vi "SpaceX Main.vi"() -> ()   [LabVIEW 2022 SP3]
uses:
  AppData/Local/Temp/703aeb86-a1ff-4ba8-9387-38d48ae470f4_SpaceX Demo.zip.0f4/SpaceX Demo/SubVIs/States.ctl
  <vilib>/LabVIEW Interface for Arduino/Type Defs/Pin Mode.ctl
panel:
  in  "Dragon Capsule Delay Time (s)":dbl=1.0 caption="Delay Time (s)"
  in  "Wave Delay (s)":dbl=1.0 caption="Delay Time (s)"
  in  "Rocket Launch Delay Time (s)":dbl caption="Delay Time (s)"
  in  "Rocket Launch Motor Pin":u8=3
  in  "Dragon Capsule Motor Pin":u8=11
  in  "Rocket Motor Speed":u8=100
  in  "Dragon Capsule Speed":u8=50
  in  "Reset Mode":bool
  in  "Rocket Backwards":bool
  in  "Capsule Backwards":bool
  out "Demo Ready?":bool
  out "Hall Effect Sensor Value":dbl
  in  "Rocket Launch Complete":bool
  in  "GO Button":bool
  in  "stop":bool
  in  "Kinect Close Button":bool
  in  "Launch Pad Pin":u8=5
  in  "Wave Pins":T1={"Wave 1 Pin"=6, "Wave 2 Pin"=7, "Wave 3 Pin"=8, "Wave 4 Pin"=9, "Wave 5"=10}
  out "State Machine: Current State":T2
  in  "Pulse Speed":u8(knob)=3 scale=1.0..10.0
  out "Launch Pad Voltage Level":dbl(knob) scale=0.0..255.0
  in  "Number of Pulses":i32=4
  in  "stop 2":bool
  # "Delay Settings"
  # "Motor Configuration"
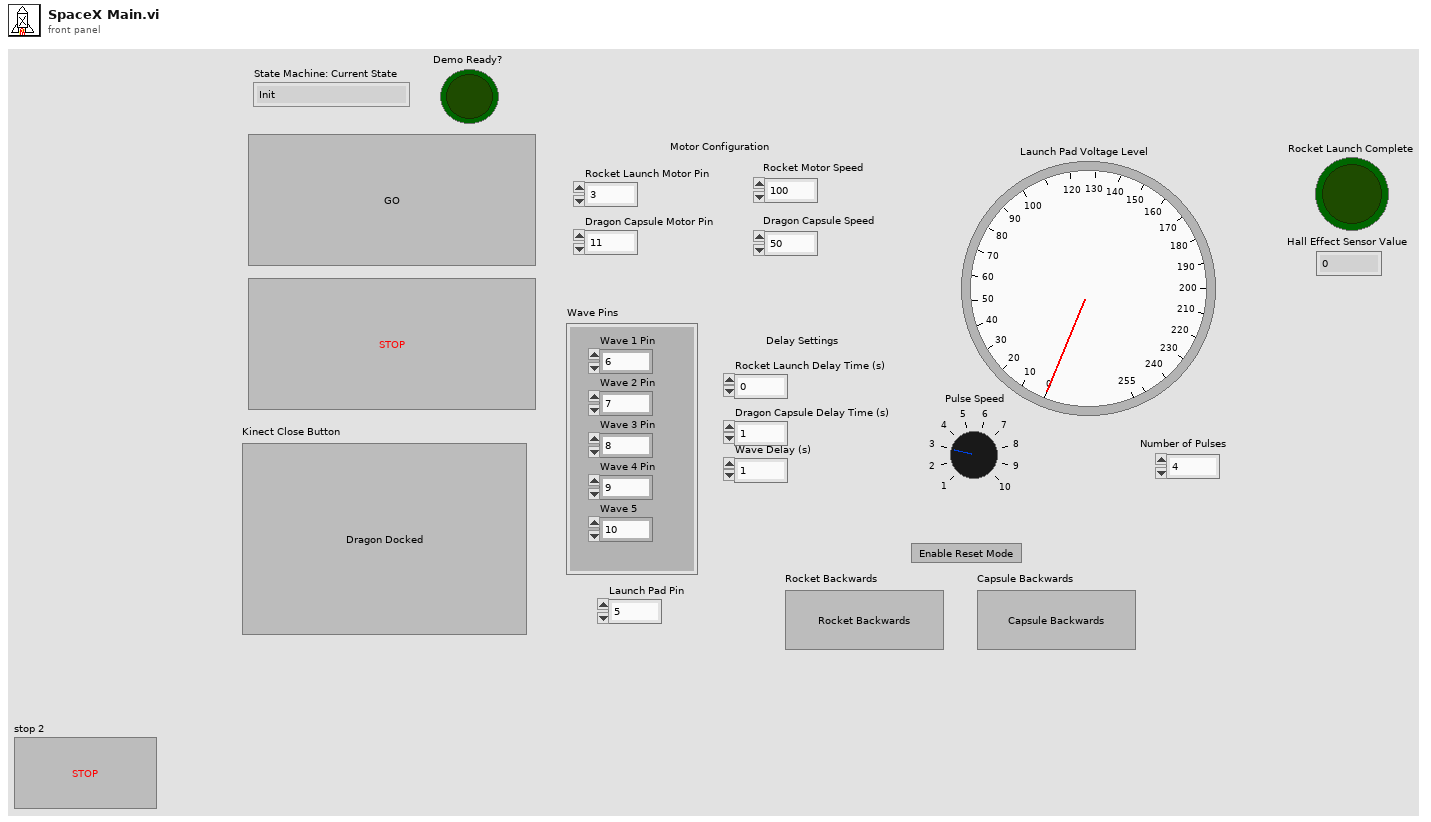
[diagram p1: front panel]
types:
  T1 = cluster{"Wave 1 Pin":u8, "Wave 2 Pin":u8, "Wave 3 Pin":u8, "Wave 4 Pin":u8, "Wave 5":u8}
  T2 = typedef "States.ctl" = enum16{"Init", "Run", "Shutdown", "Rocket Launch", "Dragon Travel", "Communicate", "Reset"}
  T3 = typedef "LabVIEW Interface for Arduino.lvlib/Pin Mode.ctl" = enum8{"Input", "Output"}
  T4 = typedef "LabVIEW Interface for Arduino.lvlib/Arduino Resource.ctl" = cluster{"VISA resource":refnum<visa-resource-name>, "Board Type":T5, "Connection Type":enum8{"USB / Serial"}, "Bytes Per Packet (15)":u8}
  T5 = typedef "LabVIEW Interface for Arduino.lvlib/Board Type.ctl" = enum16{"Uno", "Dimuelanove w/Atmega 328", "Mega 2560"}
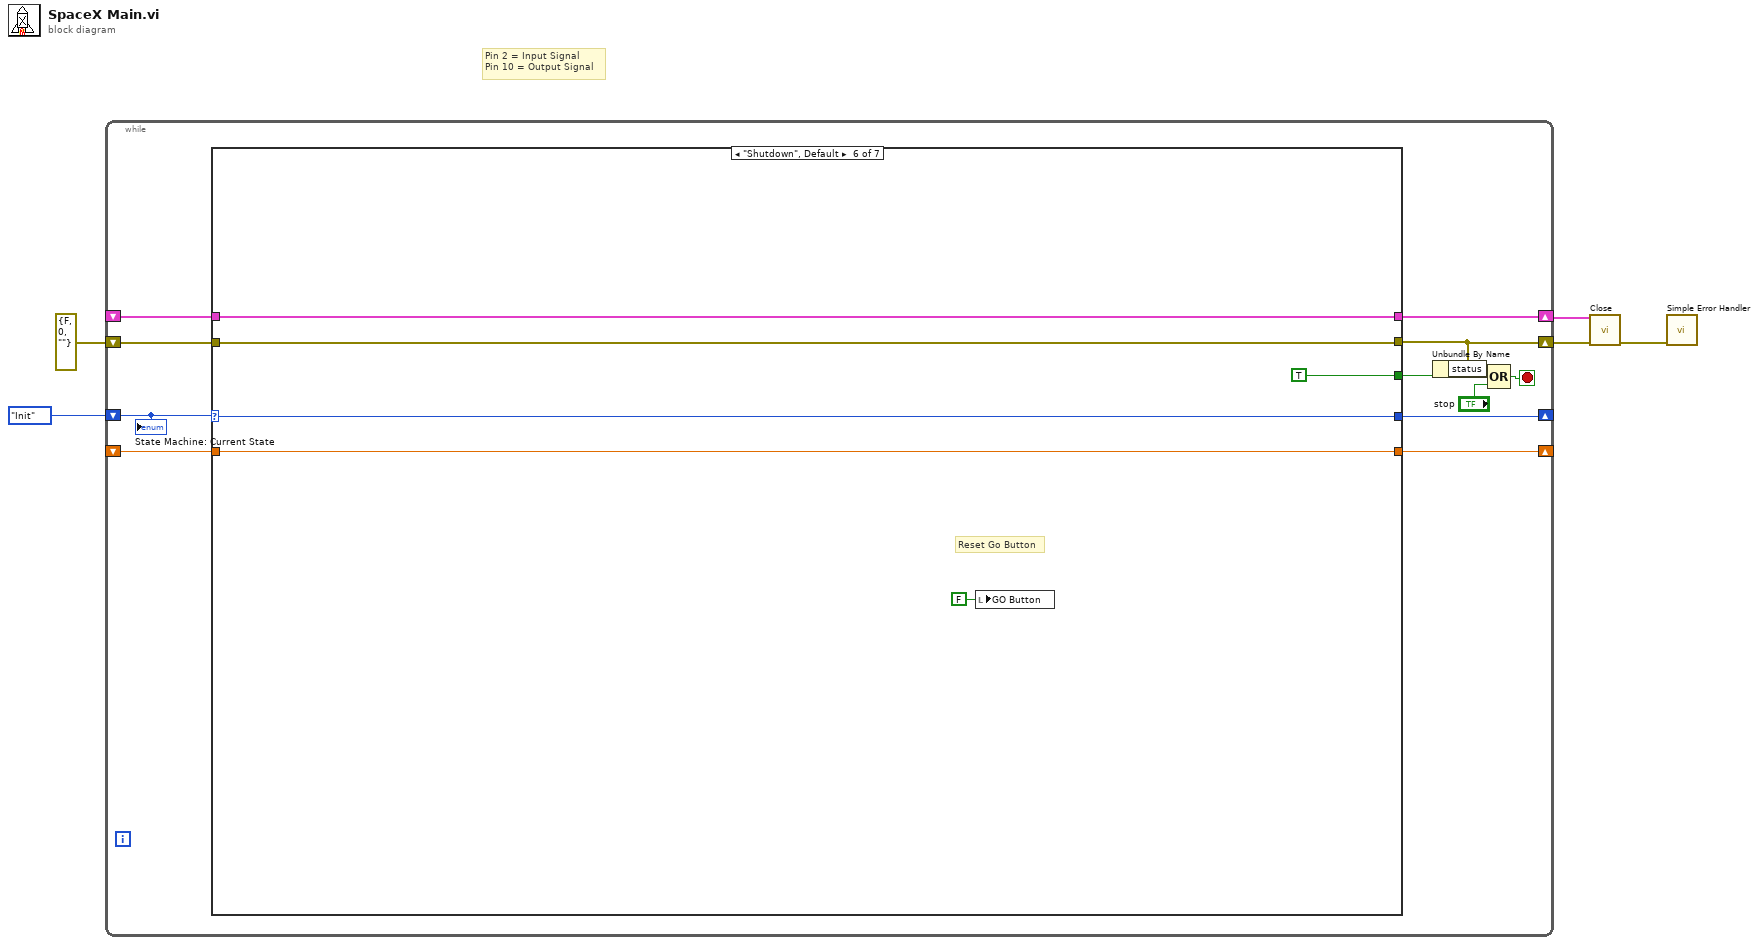
[diagram p0: block diagram]
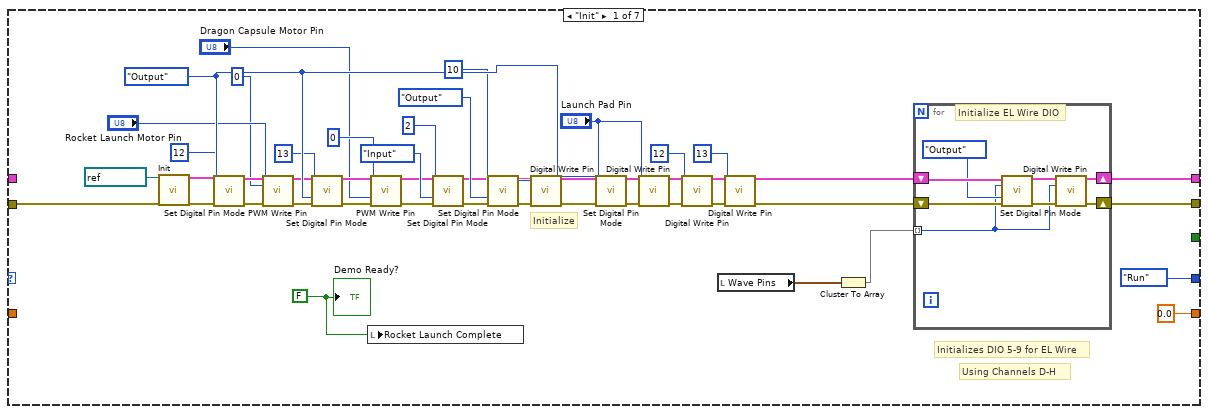
[diagram p2: hidden frame]
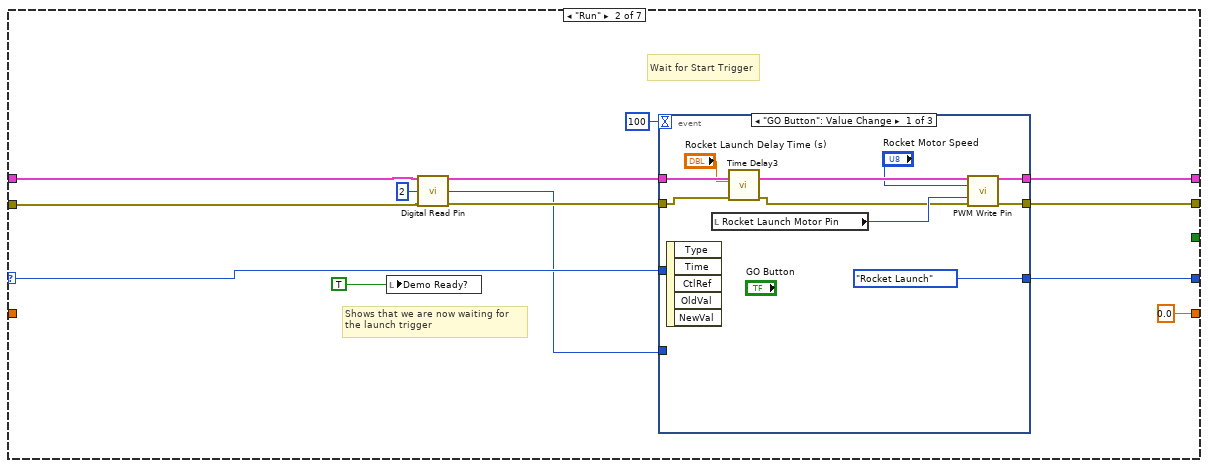
[diagram p3: hidden frame]
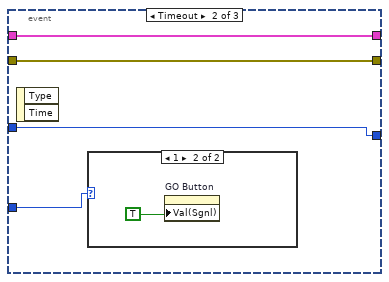
[diagram p4: hidden frame]
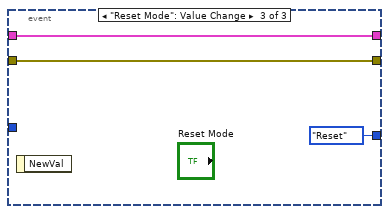
[diagram p6: hidden frame]
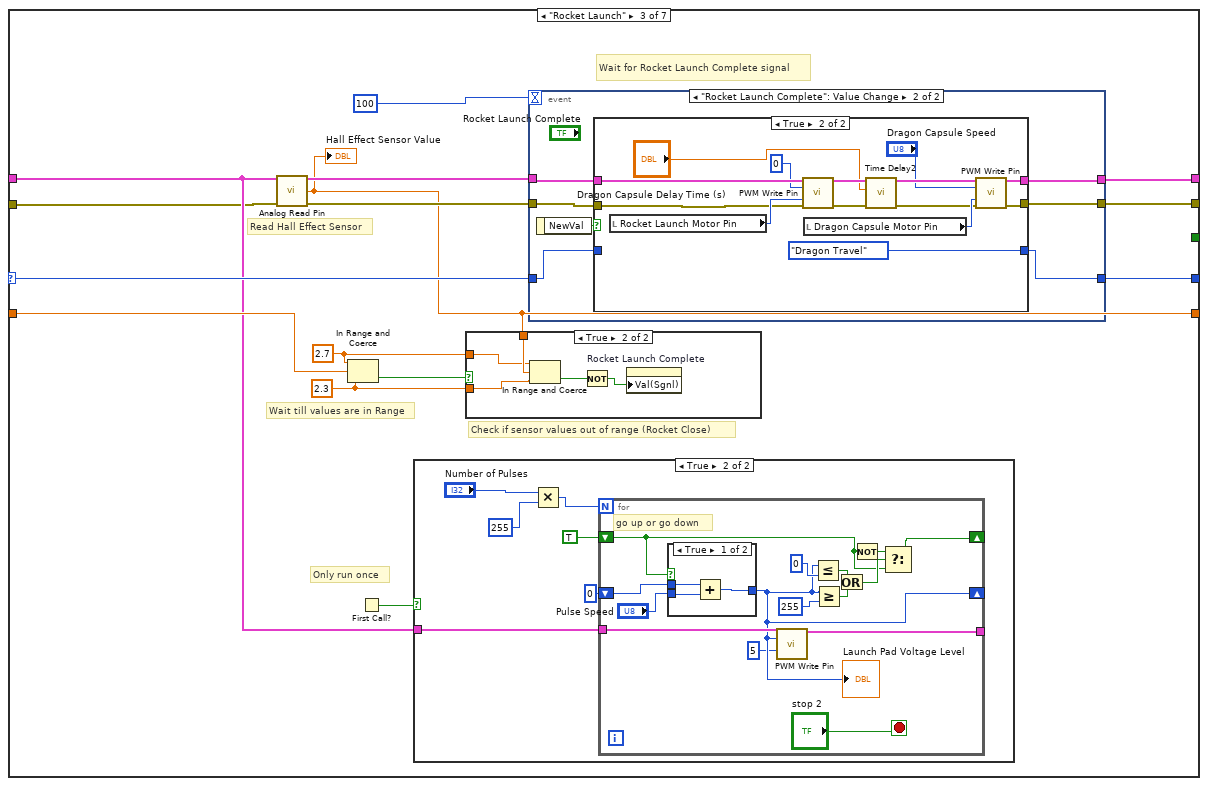
[diagram p7: hidden frame]
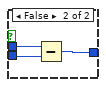
[diagram p9: hidden frame]
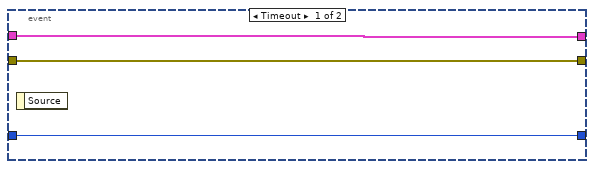
[diagram p11: hidden frame]
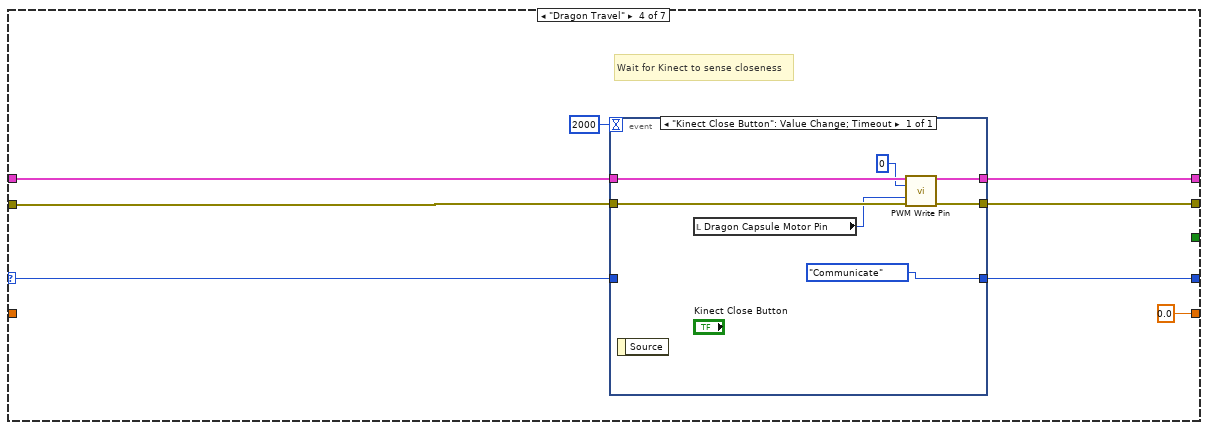
[diagram p13: hidden frame]
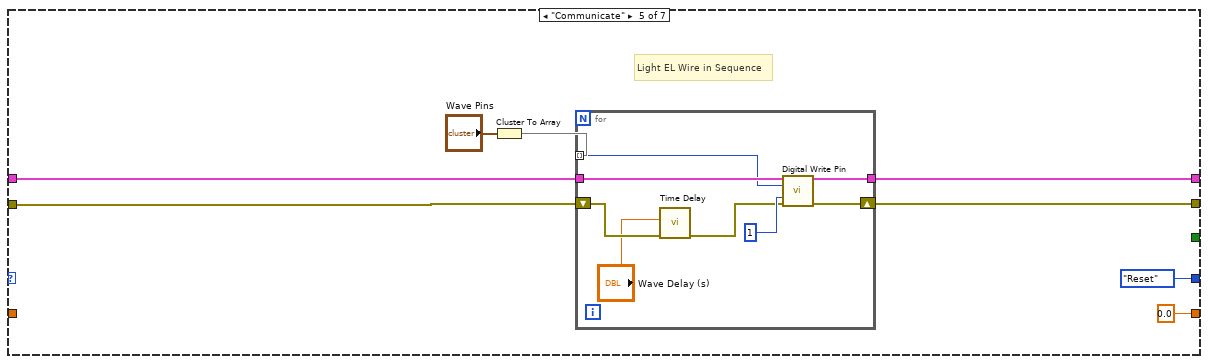
[diagram p14: hidden frame]
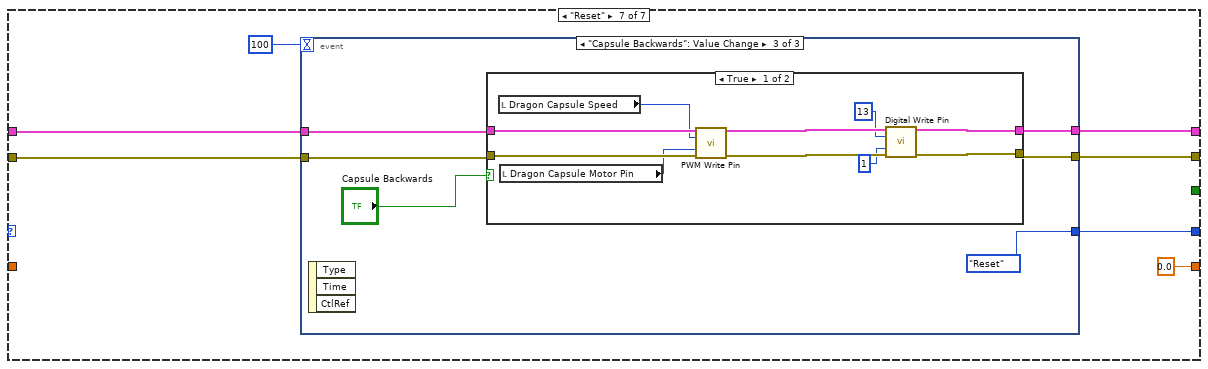
[diagram p15: hidden frame]
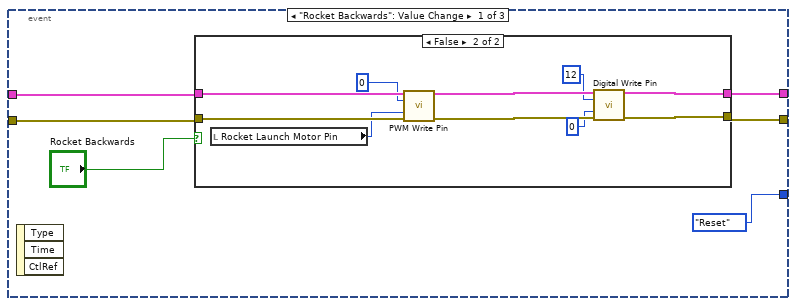
[diagram p16: hidden frame]
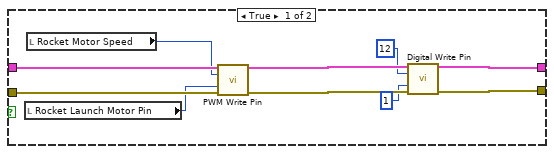
[diagram p17: hidden frame]
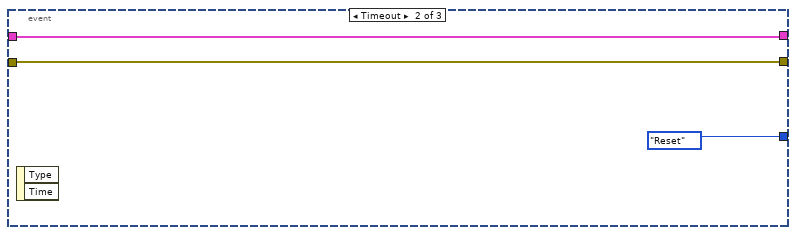
[diagram p18: hidden frame]
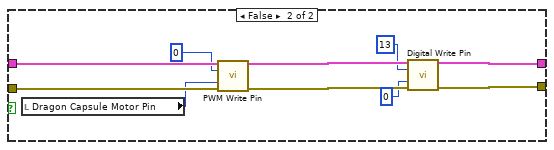
[diagram p19: hidden frame]
diagram:
  # "Pin 2 = Input Signal\nPin 10 = Output Signal"
  n1 = while {
    shift-right: [w10] -> _
    shift-left: States."Init" -> [w17]
    shift-right: [w16] -> w3
    shift-left: _ -> [w15]
    shift-right: [w11] -> w2
    shift-left: errorcluster {"status"=FALSE, "code"=0, "source"=""} ("error out") -> [w14]
    shift-right: [w9] -> _
    shift-left: _ -> [w8]
    stop <- w13 stop-if-true
    n2 = case shown="\"Shutdown\", Default" w17 {
      selector: w17 -> [_ w79 w115 w177 _ w211 _]
      tunnel: [w62 w83 w113 w180 w194 w209 w216] -> w16
      tunnel: w15 -> [_ w73 w105 w182 w196 w209 w218]
      tunnel: [w63 w82 w114 w179 w193 w208 w215] -> w11
      tunnel: w14 -> [w55 w77 w104 w181 w195 w208 w217]
      tunnel: [_ _ _ _ _ TRUE _] -> w12
      tunnel: [States."Run" w81 w117 w178 States."Reset" w211 w214] -> w10
      tunnel: [0.0 ("Voltage") 0.0 ("Voltage") w110 0.0 ("Voltage") 0.0 ("Voltage") w210 0.0 ("Voltage")] -> w9
      tunnel: w8 -> [_ _ w109 _ _ w210 _]
      frame "Init" {
        w27 = u8 10 ("Digital I/O Pin")
        w52 = Pin_Mode."Output" ("Pin Mode (Input)")
        w31 = FALSE ("Demo Ready?")
        # "Initialize"
        # "Using Channels D-H"
        # "Initializes DIO 5-9 for EL Wire"
        n3 = call <vilib>:"Init.vi"("VISA resource"=refnum<visa-resource-name> "COM3", "error in"=w55) -> ("Arduino Resource"=w54:T4, "error out"=w56:errorcluster)  [unwired: 16 in]
        n4 = call <vilib>:"Set Digital Pin Mode.vi"("Arduino Resource"=w54, "Digital I/O Pin"=u8 12, "Pin Mode (Input)"=w52, "error in"=w56) -> ("Arduino Resource"=w47:T4, "error out"=w48:errorcluster)  [unwired: 10 in]
        n5 = call <vilib>:"PWM Write Pin.vi"("Arduino Resource"=w47, "Duty Cycle (0 - 255)"=u8 0, "PWM Pin (3)"="Rocket Launch Motor Pin", "error in"=w48) -> ("Arduino Resource"=w46:T4, "error out"=w45:errorcluster)  [unwired: 10 in]
        n6 = call <vilib>:"Set Digital Pin Mode.vi"("Arduino Resource"=w46, "Digital I/O Pin"=u8 13, "Pin Mode (Input)"=w52, "error in"=w45) -> ("Arduino Resource"=w50:T4, "error out"=w51:errorcluster)  [unwired: 10 in]
        n7 = local write "Rocket Launch Complete"(w31) -> ()
        n8 = call <vilib>:"PWM Write Pin.vi"("Arduino Resource"=w50, "Duty Cycle (0 - 255)"=u8 0, "PWM Pin (3)"="Dragon Capsule Motor Pin", "error in"=w51) -> ("Arduino Resource"=w22:T4, "error out"=w21:errorcluster)  [unwired: 10 in]
        n9 = call <vilib>:"Set Digital Pin Mode.vi"("Arduino Resource"=w22, "Digital I/O Pin"=u8 2, "Pin Mode (Input)"=Pin_Mode."Input", "error in"=w21) -> ("Arduino Resource"=w24:T4, "error out"=w23:errorcluster)  [unwired: 10 in]
        n10 = call <vilib>:"Set Digital Pin Mode.vi"("Arduino Resource"=w24, "Digital I/O Pin"=w27, "Pin Mode (Input)"=Pin_Mode."Output", "error in"=w23) -> ("Arduino Resource"=w25:T4, "error out"=w26:errorcluster)  [unwired: 10 in]
        n11 = call <vilib>:"Digital Write Pin.vi"("Arduino Resource"=w25, "Digital I/O Pin (0)"=w27, "error in"=w26) -> ("Arduino Resource"=w19:T4, "error out"=w20:errorcluster)  [unwired: 11 in]
        n12 = call <vilib>:"Set Digital Pin Mode.vi"("Arduino Resource"=w19, "Digital I/O Pin"="Launch Pad Pin", "Pin Mode (Input)"=w52, "error in"=w20) -> ("Arduino Resource"=w53:T4, "error out"=w57:errorcluster)  [unwired: 10 in]
        n13 = call <vilib>:"Digital Write Pin.vi"("Arduino Resource"=w53, "Digital I/O Pin (0)"="Launch Pad Pin", "error in"=w57) -> ("Arduino Resource"=w32:T4, "error out"=w33:errorcluster)  [unwired: 11 in]
        n14 = call <vilib>:"Digital Write Pin.vi"("Arduino Resource"=w32, "Digital I/O Pin (0)"=u8 12, "error in"=w33) -> ("Arduino Resource"=w39:T4, "error out"=w38:errorcluster)  [unwired: 11 in]
        n15 = local read "Wave Pins"() -> (w60:T1)
        n16 = call <vilib>:"Digital Write Pin.vi"("Arduino Resource"=w39, "Digital I/O Pin (0)"=u8 13, "error in"=w38) -> ("Arduino Resource"=w35:T4, "error out"=w34:errorcluster)  [unwired: 11 in]
        n17 = Cluster To Array(cluster=w60) -> (array=w59:u8[])
        n18 = for {
          shift-right: [w66] -> w62
          shift-left: w35 -> [w71]
          shift-right: [w67] -> w63
          shift-left: w34 -> [w72]
          tunnel: w59 -> [w65] mode=indexing
          # "Initialize EL Wire DIO"
          n19 = call <vilib>:"Set Digital Pin Mode.vi"("Arduino Resource"=w71, "Digital I/O Pin"=w65, "Pin Mode (Input)"=Pin_Mode."Output", "error in"=w72) -> ("Arduino Resource"=w69:T4, "error out"=w68:errorcluster)  [unwired: 10 in]
          n20 = call <vilib>:"Digital Write Pin.vi"("Arduino Resource"=w69, "Digital I/O Pin (0)"=w65, "error in"=w68) -> ("Arduino Resource"=w66:T4, "error out"=w67:errorcluster)  [unwired: 11 in]
        }
        "Demo Ready?" <- w31
      }
      frame "Run" {
        # "Shows that we are now waiting for\nthe launch trigger"
        # "Wait for Start Trigger"
        n21 = local write "Demo Ready?"(TRUE ("Demo Ready?")) -> ()
        n22 = call <vilib>:"Digital Read Pin.vi"("Arduino Resource"=w73, "Digital I/O Pin (0)"=u8 2, "error in"=w77) -> ("Arduino Resource"=w78:T4, "Value"=w74:u8, "error out"=w76:errorcluster)  [unwired: 10 in]
        n23 = event shown="[0] \"GO Button\": Value Change" {
          selector: _ -> [_ _ _]
          dyn-events: _ -> [_ _ _]
          timeout: 100 -> [_ _ _]
          tunnel: w78 -> [w94 w98 w102]
          tunnel: w76 -> [w88 w97 w101]
          tunnel: [w93 w98 w102] -> w83
          tunnel: [w92 w97 w101] -> w82
          tunnel: [States."Rocket Launch" w96 States."Reset"] -> w81
          tunnel: w79 -> [_ w96 _]
          tunnel: w74 -> [_ w95 _]
          event "GO Button": Value Change {
            n24 = event-data() -> ()  [unwired: 1 in, 5 out]
            n25 = local read "Rocket Launch Motor Pin"() -> (w90:u8)
            n26 = call "Time Delay3"("error in (no error)"=w88, "Delay Time (s)"="Rocket Launch Delay Time (s)") -> ("error out"=w87:errorcluster)  [unwired: 9 in]
            n27 = call <vilib>:"PWM Write Pin.vi"("Arduino Resource"=w94, "Duty Cycle (0 - 255)"="Rocket Motor Speed", "PWM Pin (3)"=w90, "error in"=w87) -> ("Arduino Resource"=w93:T4, "error out"=w92:errorcluster)  [unwired: 10 in]
          }
          event Timeout {
            n28 = event-data() -> ()  [unwired: 1 in, 2 out]
            n29 = case shown="1" w95 {
              frame 0, Default {
              }
              frame 1 {
                n30 = property on="GO Button" class="Bool (strict)"("Val(Sgnl)"=TRUE) -> ()  [unwired: 2 in, 2 out]
              }
            }
          }
          event "Reset Mode": Value Change {
            n31 = event-data() -> ()  [unwired: 1 in, 1 out]
          }
        }
      }
      frame "Rocket Launch" {
        w106 = 2.3 ("lower limit")
        w107 = 2.7 ("upper limit")
        # "Only run once"
        # "Check if sensor values out of range (Rocket Close)"
        # "Wait till values are in Range"
        # "Read Hall Effect Sensor"
        # "Wait for Rocket Launch Complete signal"
        n32 = call <vilib>:"Analog Read Pin.vi"("Arduino Resource"=w105, "error in"=w104) -> ("Arduino Resource"=w112:T4, "Voltage"=w110:dbl, "error out"=w111:errorcluster)  [unwired: 11 in]
        "Hall Effect Sensor Value" <- w110
        n33 = In Range and Coerce(upper limit=w107, x=w109, lower limit=w106) -> (In Range?=w108:bool)  [unwired: 1 out]
        n34 = First Call?() -> (First Call?: T/F=w103:bool)
        n35 = case shown="True" w103 {
          tunnel: w105 -> [_ w118]
          frame False {
          }
          frame True {
            n36 = Multiply(x="Number of Pulses", y=255) -> (x*y=w121:i32)
            n37 = for {
              N: w121 -> [_]
              tunnel: w118 -> [w138]
              tunnel: [w137] -> _
              shift-right: [w133] -> _
              shift-left: TRUE -> [w131]
              shift-right: [w126] -> _
              shift-left: u8 0 ("PWM Pin (3)") -> [w128]
              stop <- "stop 2" stop-if-true
              # "go up or go down"
              n38 = case shown="True" w131 {
                tunnel: "Pulse Speed" -> [w141 w144]
                tunnel: w128 -> [w140 w143]
                tunnel: [w139 w142] -> w126
                frame True {
                  n39 = Add(x=w140, y=w141) -> (x+y=w139:u8)
                }
                frame False {
                  n40 = Subtract(x=w143, y=w144) -> (x-y=w142:u8)
                }
              }
              "Launch Pad Voltage Level" <- w126
              n41 = call <vilib>:"PWM Write Pin.vi"("Arduino Resource"=w138, "Duty Cycle (0 - 255)"=w126, "PWM Pin (3)"=u8 5) -> ("Arduino Resource"=w137:T4)  [unwired: 11 in, 1 out]
              n42 = Less Or Equal?(x=w126, y=u8 0 ("PWM Pin (3)")) -> (x <= y?=w136:bool)
              n43 = Greater Or Equal?(x=w126, y=u8 255 ("PWM Pin (3)")) -> (x >= y?=w135:bool)
              n44 = Or(x=w136, y=w135) -> (x .or. y?=w134:bool)
              n45 = Not(x=w131) -> (.not. x?=w132:bool)
              n46 = Select(t=w132, s=w134, f=w131) -> (s? t:f=w133:bool)
            }
          }
        }
        n47 = case shown="True" w108 {
          tunnel: w110 -> [_ w149]
          tunnel: w107 -> [_ w148]
          tunnel: w106 -> [_ w147]
          frame False {
          }
          frame True {
            n48 = In Range and Coerce(upper limit=w148, x=w149, lower limit=w147) -> (In Range?=w146:bool)  [unwired: 1 out]
            n49 = Not(x=w146) -> (.not. x?=w145:bool)
            n50 = property on="Rocket Launch Complete" class="Bool (strict)"("Val(Sgnl)"=w145) -> ()  [unwired: 2 in, 2 out]
          }
        }
        n51 = event shown="[1] \"Rocket Launch Complete\": Value Change" {
          selector: _ -> [_ _]
          dyn-events: _ -> [_ _]
          timeout: 100 -> [_ _]
          tunnel: w112 -> [w152 w159]
          tunnel: w111 -> [w151 w158]
          tunnel: [w150 w155] -> w117
          tunnel: [w151 w156] -> w114
          tunnel: [w152 w157] -> w113
          tunnel: w115 -> [w150 w153]
          event Timeout {
            n52 = event-data() -> ()  [unwired: 1 in, 1 out]
          }
          event "Rocket Launch Complete": Value Change {
            n53 = event-data() -> ("NewVal"=w154:bool)  [unwired: 1 in]
            n54 = case shown="True" w154 {
              tunnel: w159 -> [w161 w175]
              tunnel: w158 -> [w162 w166]
              tunnel: [w161 w173] -> w157
              tunnel: [w162 w172] -> w156
              tunnel: [w160 States."Dragon Travel"] -> w155
              tunnel: w153 -> [w160 _]
              frame False {
              }
              frame True {
                n55 = local read "Rocket Launch Motor Pin"() -> (w168:u8)
                n56 = call <vilib>:"PWM Write Pin.vi"("Arduino Resource"=w175, "Duty Cycle (0 - 255)"=u8 0, "PWM Pin (3)"=w168, "error in"=w166) -> ("Arduino Resource"=w171:T4, "error out"=w165:errorcluster)  [unwired: 10 in]
                n57 = local read "Dragon Capsule Motor Pin"() -> (w170:u8)
                n58 = call "Time Delay2"("error in (no error)"=w165, "Delay Time (s)"="Dragon Capsule Delay Time (s)") -> ("error out"=w164:errorcluster)  [unwired: 9 in]
                n59 = call <vilib>:"PWM Write Pin.vi"("Arduino Resource"=w171, "Duty Cycle (0 - 255)"="Dragon Capsule Speed", "PWM Pin (3)"=w170, "error in"=w164) -> ("Arduino Resource"=w173:T4, "error out"=w172:errorcluster)  [unwired: 10 in]
              }
            }
          }
        }
      }
      frame "Dragon Travel" {
        # "Wait for Kinect to sense closeness"
        n60 = event shown="[0] \"Kinect Close Button\": Value Change;  Timeout" {
          selector: _ -> [_]
          dyn-events: _ -> [_]
          timeout: 2000 -> [_]
          tunnel: w182 -> [w190]
          tunnel: w181 -> [w189]
          tunnel: [w185] -> w180
          tunnel: [w186] -> w179
          tunnel: [States."Communicate"] -> w178
          tunnel: w177 -> [_]
          event "Kinect Close Button": Value Change; Timeout {
            n61 = event-data() -> ()  [unwired: 1 in, 1 out]
            n62 = local read "Dragon Capsule Motor Pin"() -> (w187:u8)
            n63 = call <vilib>:"PWM Write Pin.vi"("Arduino Resource"=w190, "Duty Cycle (0 - 255)"=u8 0, "PWM Pin (3)"=w187, "error in"=w189) -> ("Arduino Resource"=w185:T4, "error out"=w186:errorcluster)  [unwired: 10 in]
          }
        }
      }
      frame "Communicate" {
        # "Light EL Wire in Sequence"
        n64 = Cluster To Array(cluster="Wave Pins") -> (array=w197:u8[])
        n65 = for {
          tunnel: w197 -> [w202] mode=indexing
          tunnel: w196 -> [w203]
          tunnel: [w201] -> w194
          shift-right: [w200] -> w193
          shift-left: w195 -> [w204]
          n66 = call "Time Delay"("error in (no error)"=w204, "Delay Time (s)"="Wave Delay (s)") -> ("error out"=w205:errorcluster)  [unwired: 9 in]
          n67 = call <vilib>:"Digital Write Pin.vi"("Arduino Resource"=w203, "Digital I/O Pin (0)"=w202, "Value (0)"=u8 1, "error in"=w205) -> ("Arduino Resource"=w201:T4, "error out"=w200:errorcluster)  [unwired: 10 in]
        }
      }
      frame "Shutdown", Default {
        # "Reset Go Button"
        n68 = local write "GO Button"(FALSE ("GO Button")) -> ()
      }
      frame "Reset" {
        n69 = event shown="[2] \"Capsule Backwards\": Value Change" {
          selector: _ -> [_ _ _]
          dyn-events: _ -> [_ _ _]
          timeout: 100 -> [_ _ _]
          tunnel: w218 -> [w225 w248 w254]
          tunnel: w217 -> [w224 w247 w253]
          tunnel: [w223 w248 w252] -> w216
          tunnel: [w222 w247 w251] -> w215
          tunnel: [States."Reset" States."Reset" States."Reset"] -> w214
          event "Rocket Backwards": Value Change {
            n70 = event-data() -> ()  [unwired: 1 in, 3 out]
            n71 = case shown="False" "Rocket Backwards" {
              tunnel: w225 -> [w235 w245]
              tunnel: w224 -> [w234 w244]
              tunnel: [w231 w242] -> w223
              tunnel: [w230 w241] -> w222
              frame True {
                n72 = local read "Rocket Launch Motor Pin"() -> (w233:u8)
                n73 = local read "Rocket Motor Speed"() -> (w232:u8)
                n74 = call <vilib>:"PWM Write Pin.vi"("Arduino Resource"=w235, "Duty Cycle (0 - 255)"=w232, "PWM Pin (3)"=w233, "error in"=w234) -> ("Arduino Resource"=w228:T4, "error out"=w229:errorcluster)  [unwired: 10 in]
                n75 = call <vilib>:"Digital Write Pin.vi"("Arduino Resource"=w228, "Digital I/O Pin (0)"=u8 12, "Value (0)"=u8 1, "error in"=w229) -> ("Arduino Resource"=w231:T4, "error out"=w230:errorcluster)  [unwired: 10 in]
              }
              frame False {
                n76 = local read "Rocket Launch Motor Pin"() -> (w243:u8)
                n77 = call <vilib>:"PWM Write Pin.vi"("Arduino Resource"=w245, "Duty Cycle (0 - 255)"=u8 0, "PWM Pin (3)"=w243, "error in"=w244) -> ("Arduino Resource"=w239:T4, "error out"=w240:errorcluster)  [unwired: 10 in]
                n78 = call <vilib>:"Digital Write Pin.vi"("Arduino Resource"=w239, "Digital I/O Pin (0)"=u8 12, "Value (0)"=u8 0, "error in"=w240) -> ("Arduino Resource"=w242:T4, "error out"=w241:errorcluster)  [unwired: 10 in]
              }
            }
          }
          event Timeout {
            n79 = event-data() -> ()  [unwired: 1 in, 2 out]
          }
          event "Capsule Backwards": Value Change {
            n80 = event-data() -> ()  [unwired: 1 in, 3 out]
            n81 = case shown="True" "Capsule Backwards" {
              tunnel: w254 -> [w264 w274]
              tunnel: w253 -> [w263 w273]
              tunnel: [w260 w271] -> w252
              tunnel: [w259 w270] -> w251
              frame True {
                n82 = local read "Dragon Capsule Speed"() -> (w261:u8)
                n83 = local read "Dragon Capsule Motor Pin"() -> (w262:u8)
                n84 = call <vilib>:"PWM Write Pin.vi"("Arduino Resource"=w264, "Duty Cycle (0 - 255)"=w261, "PWM Pin (3)"=w262, "error in"=w263) -> ("Arduino Resource"=w257:T4, "error out"=w258:errorcluster)  [unwired: 10 in]
                n85 = call <vilib>:"Digital Write Pin.vi"("Arduino Resource"=w257, "Digital I/O Pin (0)"=u8 13, "Value (0)"=u8 1, "error in"=w258) -> ("Arduino Resource"=w260:T4, "error out"=w259:errorcluster)  [unwired: 10 in]
              }
              frame False {
                n86 = local read "Dragon Capsule Motor Pin"() -> (w272:u8)
                n87 = call <vilib>:"PWM Write Pin.vi"("Arduino Resource"=w274, "Duty Cycle (0 - 255)"=u8 0, "PWM Pin (3)"=w272, "error in"=w273) -> ("Arduino Resource"=w268:T4, "error out"=w269:errorcluster)  [unwired: 10 in]
                n88 = call <vilib>:"Digital Write Pin.vi"("Arduino Resource"=w268, "Digital I/O Pin (0)"=u8 13, "Value (0)"=u8 0, "error in"=w269) -> ("Arduino Resource"=w271:T4, "error out"=w270:errorcluster)  [unwired: 10 in]
              }
            }
          }
        }
      }
    }
    n89 = Unbundle By Name(w11) -> ("status"=w6:bool)
    n90 = Compound Arithmetic op=OR(w6, w12, "stop") -> (w13:bool)
    "State Machine: Current State" <- w17
  }
  n91 = call <vilib>:"Close.vi"("Arduino Resource"=w3, "error in"=w2) -> ("error out"=w1:errorcluster)  [unwired: 13 in]
  n92 = call <vilib>:"Simple Error Handler.vi"("error in (no error)"=w1) -> ()  [unwired: 4 in, 5 out]
